vi "DiffOdometry_Update.vi"(8 "Reset":bool, 9 "Heading":T1={"VALUE"=0.0, "COS"=1.0, "SIN"=0.0}, 10 "RightDistance":dbl, 11 "LeftDistance":dbl) -> (3 "CurrentRelativePose":T2)   [LabVIEW 2019, in "PathExecution_Library.lvlib"]
doc: "Class for differential drive odometry. Odometry allows you to track the robot's position on the field over the course of a match using readings from 2 encoders and a gyroscope.\n\nTeams can use odometry during the autonomous period for complex tasks like path following. Furthermore, odometry can be used for latency compensation when using computer-vision systems.\n\nUpdates the robot position on the field using distance measurements from encoders. This method is more numerically accurate than using velocities to integrate the pose and is also advantageous for teams that are using lower CPR encoders."
uses:
  PathExecution_Library.lvlib
  POSE.ctl
  TRANSLATION.ctl
  ROTATION.ctl
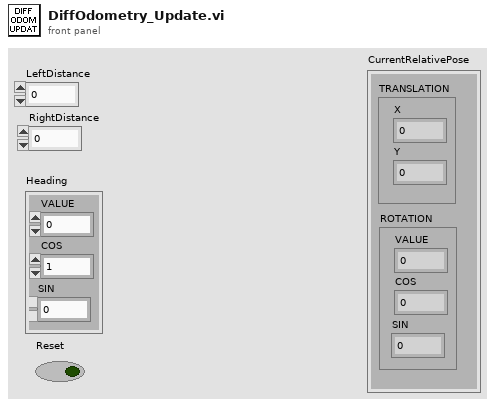
[diagram p1: front panel]
types:
  T1 = typedef "PathExecution_Library.lvlib/ROTATION.ctl" = cluster{"VALUE":dbl, "COS":dbl, "SIN":dbl}
  T2 = typedef "PathExecution_Library.lvlib/POSE.ctl" = cluster{"TRANSLATION":T3, "ROTATION":T1}
  T3 = typedef "PathExecution_Library.lvlib/TRANSLATION.ctl" = cluster{"X":dbl, "Y":dbl}
  T4 = typedef "PathExecution_Library.lvlib/TWIST.ctl" = cluster{"dX":dbl, "dY":dbl, "dTHETA":dbl}
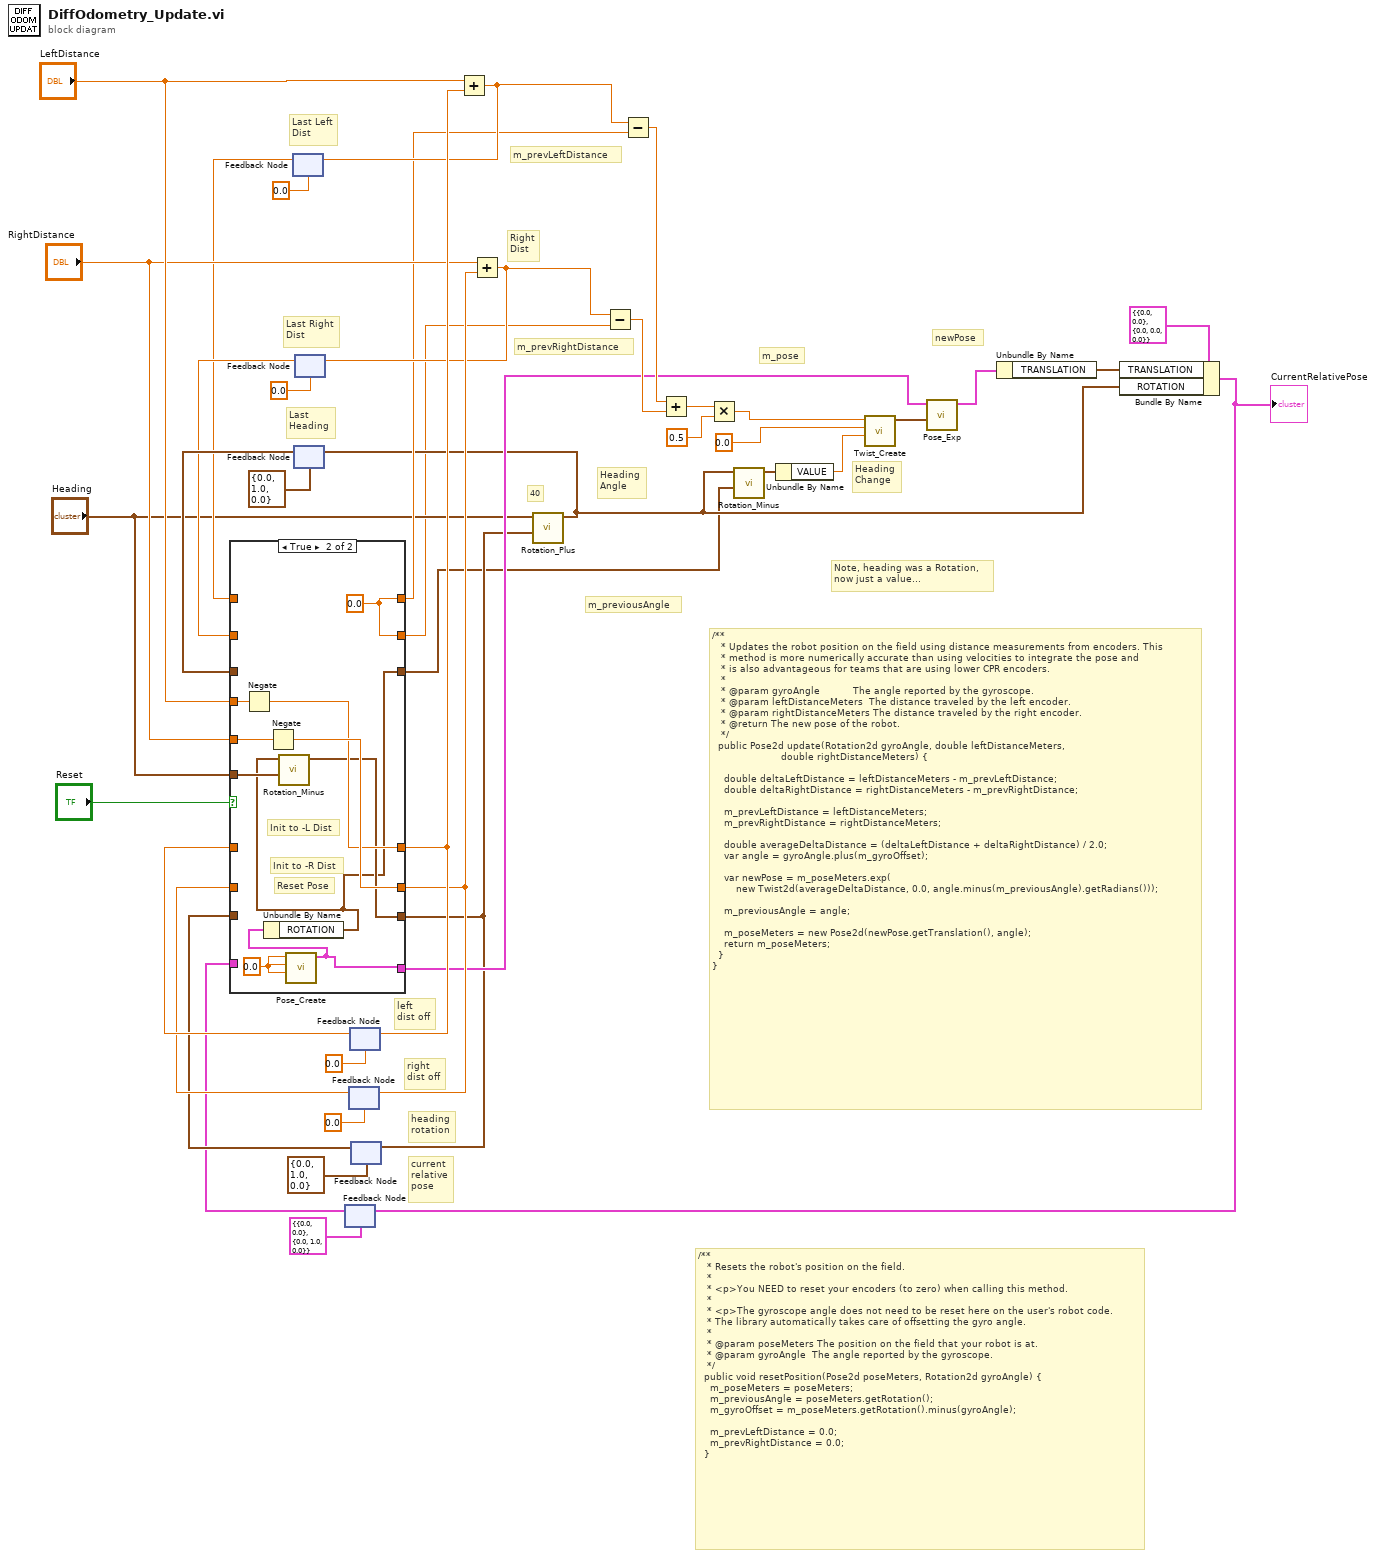
[diagram p0: block diagram]
diagram:
  # "40"
  # "left\ndist off"
  # "right\ndist off"
  # "heading\nrotation"
  # "current \nrelative\npose"
  # "/**\n   * Resets the robot's position on the field.\n   *\n   * <p>You NEED to reset your encoders (to zero) when calling this method.\n   *\n   * <p>The gyroscope angle does not need to be reset here on the user's robot code.\n   * The library automatically takes care of offsetting the gyro angle.\n   *\n   * @param poseMeters The position on the field that your robot is at.\n   * @param gyroAngle  The angle reported by the gyroscope.\n   */\n  public void resetPosition(Pose2d poseMeters, Rotation2d gyroAngle) {\n    m_poseMeters = poseMeters;\n    m_previousAngle = poseMeters.getRotation();\n    m_gyroOffset = m_poseMeters.getRotation().minus(gyroAngle);\n\n    m_prevLeftDistance = 0.0;\n    m_prevRightDistance = 0.0;\n  }"
  # "Heading\nChange"
  # "Note, heading was a Rotation,\nnow just a value..."
  # "Last\nHeading"
  # "Last Right\nDist"
  # "Last Left\nDist"
  # "Right\nDist"
  # "/**\n   * Updates the robot position on the field using distance measurements from encoders. This\n   * method is more numerically accurate than using velocities to integrate the pose and\n   * is also advantageous for teams that are using lower CPR encoders.\n   *\n   * @param gyroAngle           The angle reported by the gyroscope.\n   * @param leftDistanceMeters  The distance traveled by the left encoder.\n   * @param rightDistanceMeters The distance traveled by the right encoder.\n   * @return The new pose of the robot.\n   */\n  public Pose2d update(Rotation2d gyroAngle, double leftDistanceMeters,\n                       double rightDistanceMeters) {\n\n    double deltaLeftDistance = leftDistanceMeters - m_prevLeftDistance;\n    double deltaRightDistance = rightDistanceMeters - m_prevRightDistance;\n\n    m_prevLeftDistance = leftDistanceMeters;\n    m_prevRightDistance = rightDistanceMeters;\n\n    double averageDeltaDistance = (deltaLeftDistance + deltaRightDistance) / 2.0;\n    var angle = gyroAngle.plus(m_gyroOffset);\n\n    var newPose = m_poseMeters.exp(\n        new Twist2d(averageDeltaDistance, 0.0, angle.minus(m_previousAngle).getRadians()));\n\n    m_previousAngle = angle;\n\n    m_poseMeters = new Pose2d(newPose.getTranslation(), angle);\n    return m_poseMeters;\n  }\n}"
  # "newPose"
  # "Heading\nAngle"
  # "m_prevRightDistance"
  # "m_prevLeftDistance"
  # "m_previousAngle"
  # "m_pose"
  n1 = feedback #1(0.0 ("LeftDistance")) -> (w14:dbl)
  n2 = feedback #2(T1 {"VALUE"=0.0, "COS"=1.0, "SIN"=0.0} ("ROTATION")) -> (w17:T1)
  n3 = feedback #3(0.0 ("RightDistance")) -> (w16:dbl)
  n4 = feedback #4(T2 {"TRANSLATION"={"X"=0.0, "Y"=0.0}, "ROTATION"={"VALUE"=0.0, "COS"=1.0, "SIN"=0.0}} ("POSE")) -> (w19:T2)
  n5 = feedback #5(0.0 ("LeftDistance")) -> (w33:dbl)
  n6 = feedback #6(0.0 ("LeftDistance")) -> (w34:dbl)
  n7 = feedback #7(T1 {"VALUE"=0.0, "COS"=1.0, "SIN"=0.0} ("ROTATION")) -> (w32:T1)
  n8 = case shown="True" "Reset" {
    tunnel: "Heading" -> [_ w53]
    tunnel: "RightDistance" -> [_ w57]
    tunnel: "LeftDistance" -> [_ w58]
    tunnel: [w48 w55] -> w28
    tunnel: [w47 w56] -> w24
    tunnel: [w46 w54] -> w4
    tunnel: w34 -> [w48 _]
    tunnel: w33 -> [w47 _]
    tunnel: w32 -> [w46 _]
    tunnel: [w45 w51] -> w18
    tunnel: w19 -> [w45 _]
    tunnel: w17 -> [w44 _]
    tunnel: [w44 w50] -> w2
    tunnel: w16 -> [w43 _]
    tunnel: [w43 w49] -> w1
    tunnel: [w42 w49] -> w15
    tunnel: w14 -> [w42 _]
    frame False {
      # "Last Left Dist"
      # "Last Right Dist"
      # "Last Heading"
      # "(-) Left Dist at Reset"
      # "(-) Right Dist at Reset"
      # "Heading at Reset"
      # "Saved Relative POSE"
    }
    frame True {
      w49 = 0.0 ("LeftDistance")
      w52 = 0.0 ("X")
      # "Init to -L Dist"
      # "Init to -R Dist"
      # "Reset Pose"
      n9 = Negate(x=w58) -> (-x=w55:dbl)
      n10 = Negate(x=w57) -> (-x=w56:dbl)
      n11 = call "Pose_Create.vi"("Heading"=w52, "Y"=w52, "X"=w52) -> ("out POSe"=w51:T2)  [unwired: 8 in]
      n12 = Unbundle By Name(w51) -> ("ROTATION"=w50:T1)
      n13 = call "Rotation_Minus.vi"("other ROTATION"=w53, "in ROTATION"=w50) -> ("out ROTATION"=w54:T1)  [unwired: 9 in]
    }
  }
  n14 = feedback-in #5(w24) -> ()
  n15 = feedback-in #6(w28) -> ()
  n16 = feedback-in #7(w4) -> ()
  n17 = Add(x="LeftDistance", y=w28) -> (x+y=w26:dbl)
  n18 = feedback-in #1(w26) -> ()
  n19 = Add(x="RightDistance", y=w24) -> (x+y=w23:dbl)
  n20 = feedback-in #3(w23) -> ()
  n21 = call "Rotation_Plus.vi"("other ROTATION"=w4, "in ROTATION"="Heading") -> ("out ROTATION"=w3:T1)  [unwired: 9 in]
  n22 = feedback-in #2(w3) -> ()
  n23 = Subtract(x=w23, y=w1) -> (x-y=w40:dbl)
  n24 = Subtract(x=w26, y=w15) -> (x-y=w41:dbl)
  n25 = Add(x=w41, y=w40) -> (x+y=w39:dbl)
  n26 = Multiply(x=w39, y=0.5) -> (x*y=w22:dbl)
  n27 = call "Rotation_Minus.vi"("other ROTATION"=w2, "in ROTATION"=w3) -> ("out ROTATION"=w9:T1)  [unwired: 9 in]
  n28 = Unbundle By Name(w9) -> ("VALUE"=w8:dbl)
  n29 = call "Twist_Create.vi"("dTHETA"=w8, "dY"=0.0 ("DeltaY"), "dX"=w22) -> ("TWIST"=w20:T4)  [unwired: 8 in]
  n30 = call "Pose_Exp.vi"("TWIST"=w20, "POSE"=w18) -> ("UpdatedPose"=w13:T2)  [unwired: 9 in]
  n31 = Unbundle By Name(w13) -> ("TRANSLATION"=w11:T3)
  n32 = Bundle By Name(cluster=T2 {"TRANSLATION"={"X"=0.0, "Y"=0.0}, "ROTATION"={"VALUE"=0.0, "COS"=0.0, "SIN"=0.0}} ("POSE"), "TRANSLATION"=w11, "ROTATION"=w3) -> (w10:T2)
  "CurrentRelativePose" <- w10
  n33 = feedback-in #4(w10) -> ()
